vi "Esporta generiche.vi"(4 "Foglio Dati":string, 5 "Array":string[][](array[string]), 6 "Array in":string[][](array[string]), 7 "Nomi colonne":string[](array[string]), 8 "error in (no error)":errorcluster, 9 "sep. decimale numeri esportati":enum16{"Virgola", "Punto"}(ring), 10 "Nome fogli":T1(array[cluster]), 11 "NI_report in":refnum<class "NI_report.lvclass">) -> (0 "error out":errorcluster, 2 "Prova presente":bool, 3 "NI_report out":refnum<class "NI_report.lvclass">)   [LabVIEW 2019]
uses:
  <vilib>/Utility/NIReport.llb/NI_report.lvclass
  <vilib>/addons/_office/excel.llb/Excel Easy Table (str).vi
  <vilib>/addons/_office/NI_ReportGenerationToolkit.lvlib
  <vilib>/Utility/NIReport.llb/Excel/NI_Excel.lvclass
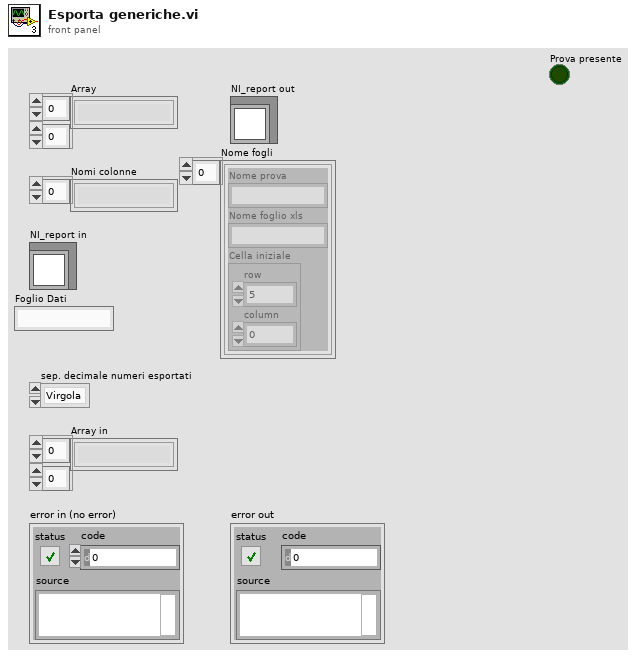
[diagram p1: front panel]
types:
  T1 = cluster{"Nome prova":string, "Nome foglio xls":string, "Cella iniziale":cluster{"row":i32, "column":i32}}[]
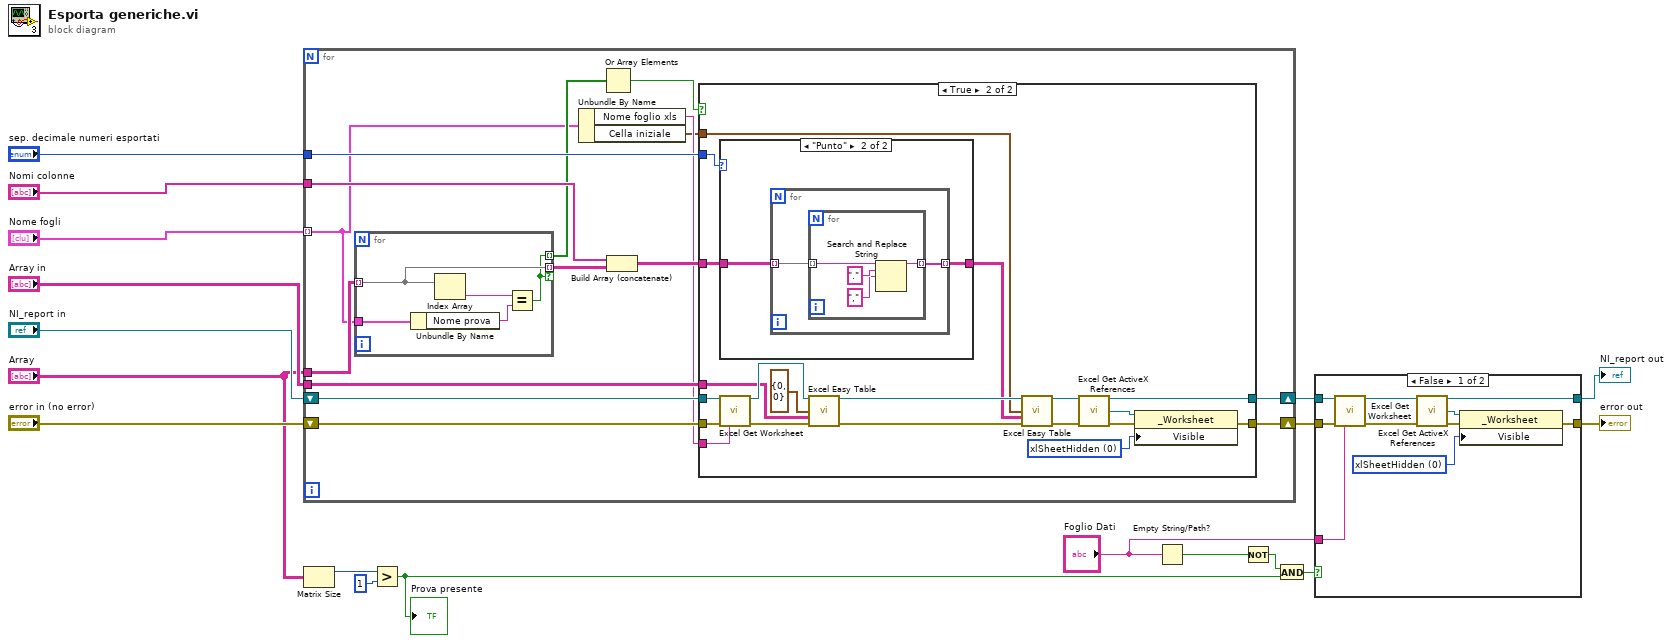
[diagram p0: block diagram]
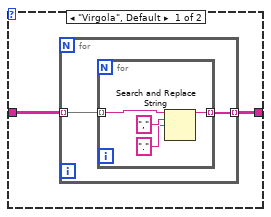
[diagram p4: hidden frame]
diagram:
  n1 = for {
    tunnel: "Array" -> [w33]
    tunnel: "Nome fogli" -> [w21] mode=indexing
    shift-right: [w27] -> w9
    shift-left: "NI_report in" -> [w30]
    shift-right: [w26] -> w7
    shift-left: "error in (no error)" -> [w29]
    tunnel: "Nomi colonne" -> [w32]
    tunnel: "Array in" -> [w28]
    tunnel: "sep. decimale numeri esportati" -> [w24]
    n2 = for {
      tunnel: w33 -> [w75] mode=indexing
      tunnel: w21 -> [w74]
      tunnel: [w75] -> w31 mode=indexing if=w72
      tunnel: [w72] -> w23 mode=indexing
      n3 = Unbundle By Name(w74) -> ("Nome prova"=w73:string)
      n4 = Index Array(array=w75) -> (element=w76:string)  [unwired: 1 in]
      n5 = Equal?(x=w76, y=w73) -> (x = y?=w72:bool)
    }
    n6 = Unbundle By Name(w21) -> ("Nome foglio xls"=w20:string, "Cella iniziale"=w19:cluster{"row":i32, "column":i32})
    n7 = Or Array Elements(Boolean array=w23) -> (logical OR=w22:bool)
    n8 = Build Array (concatenate)(w32, w31) -> (w25:string[][])
    n9 = case shown="True" w22 {
      tunnel: w30 -> [w35 w53]
      tunnel: w29 -> [w34 w51]
      tunnel: w28 -> [_ w49]
      tunnel: [w35 w38] -> w27
      tunnel: [w34 w37] -> w26
      tunnel: w25 -> [_ w36]
      tunnel: w24 -> [_ w46]
      tunnel: w20 -> [_ w45]
      tunnel: w19 -> [_ w44]
      frame False {
      }
      frame True {
        w42 = 0 items=["xlSheetVisible"=-1, "xlSheetHidden"=0, "xlSheetVeryHidden"=2] ("Visible")
        n10 = case shown="\"Punto\"" w46 {
          tunnel: w36 -> [w57 w65]
          tunnel: [w56 w64] -> w47
          frame "Virgola", Default {
            n11 = for {
              tunnel: w57 -> [w59] mode=indexing
              tunnel: [w58] -> w56 mode=indexing
              n12 = for {
                tunnel: w59 -> [w63] mode=indexing
                tunnel: [w60] -> w58 mode=indexing
                n13 = Search and Replace String(input string=w63, search string=",", replace string="." ("search string")) -> (result string=w60:string)  [unwired: 5 in, 3 out]
              }
            }
          }
          frame "Punto" {
            n14 = for {
              tunnel: w65 -> [w67] mode=indexing
              tunnel: [w66] -> w64 mode=indexing
              n15 = for {
                tunnel: w67 -> [w71] mode=indexing
                tunnel: [w68] -> w66 mode=indexing
                n16 = Search and Replace String(input string=w71, search string=".", replace string="," ("search string")) -> (result string=w68:string)  [unwired: 5 in, 3 out]
              }
            }
          }
        }
        n17 = call <vilib>:"Excel Get Worksheet.vi"("report in"=w53, "error in (no error)"=w51, "name (\"\")"=w45) -> ("report out"=w52:refnum<class "NI_report.lvclass">, "error out"=w50:errorcluster)  [unwired: 11 in]
        n18 = call-poly <vilib>:"Excel Easy Table.vi"("report in"=w52, "start (0, 0)"=cluster{"row":i32, "column":i32} {"row"=0, "column"=0}, "text data"=w49, "error in (no error)"=w50) -> ("report out"=w55:refnum<class "NI_report.lvclass">, "error out"=w54:errorcluster)  [unwired: 7 in, 3 out]
        n19 = call-poly <vilib>:"Excel Easy Table.vi"("report in"=w55, "start (0, 0)"=w44, "text data"=w47, "error in (no error)"=w54) -> ("report out"=w40:refnum<class "NI_report.lvclass">, "error out"=w39:errorcluster)  [unwired: 7 in, 3 out]
        n20 = call <vilib>:"Excel Get ActiveX References.vi"("report in"=w40, "error in (no error)"=w39) -> ("report out"=w38:refnum<class "NI_report.lvclass">, "Excel._Worksheet"=w43:refnum<k7>, "error out"=w41:errorcluster)  [unwired: 7 in, 4 out]
        n21 = property on="Property Node" class="_Worksheet"(reference=w43, error in=w41, "Visible"=w42) -> (error out=w37:errorcluster)  [unwired: 1 out]
      }
    }
  }
  n22 = Matrix Size(0:"Array") -> (1:w13:i32)  [unwired: 1 out]
  n23 = Greater?(x=w13, y=1) -> (0:w5:bool)
  "Prova presente" <- w5
  n24 = Empty String/Path?(string/path="Foglio Dati") -> (empty?=w3:bool)
  n25 = Not(x=w3) -> (.not. x?=w1:bool)
  n26 = And(x=w1, y=w5) -> (x .and. y?=w2:bool)
  n27 = case shown="False" w2 {
    tunnel: w9 -> [w86 w87]
    tunnel: w7 -> [w81 w88]
    tunnel: [w80 w88] -> w6
    tunnel: [w78 w87] -> w8
    tunnel: "Foglio Dati" -> [w77 _]
    frame False {
      w85 = 0 items=["xlSheetVisible"=-1, "xlSheetHidden"=0, "xlSheetVeryHidden"=2] ("Visible")
      n28 = call <vilib>:"Excel Get Worksheet.vi"("report in"=w86, "error in (no error)"=w81, "name (\"\")"=w77) -> ("report out"=w83:refnum<class "NI_report.lvclass">, "error out"=w82:errorcluster)  [unwired: 11 in]
      n29 = call <vilib>:"Excel Get ActiveX References.vi"("report in"=w83, "error in (no error)"=w82) -> ("report out"=w78:refnum<class "NI_report.lvclass">, "Excel._Worksheet"=w79:refnum<k7>, "error out"=w84:errorcluster)  [unwired: 7 in, 4 out]
      n30 = property on="Property Node" class="_Worksheet"(reference=w79, error in=w84, "Visible"=w85) -> (error out=w80:errorcluster)  [unwired: 1 out]
    }
    frame True {
    }
  }
  "error out" <- w6
  "NI_report out" <- w8
